vi "rosbridge.vi"(11 "ROS IP":string) -> (3 "incomming\nmessage":T1)   [LabVIEW 2013]
panel:
  out "connected?":bool
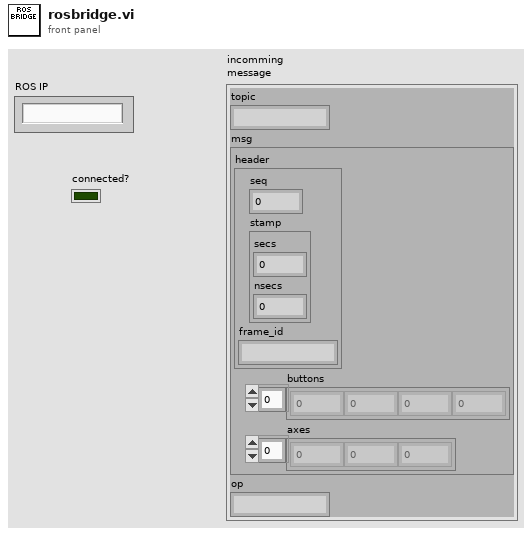
[diagram p1: front panel]
types:
  T1 = cluster{"topic":string, "msg":cluster{"header":cluster{"seq":u32, "stamp":cluster{"secs":u32, "nsecs":i32}, "frame_id":string}, "buttons":i32[], "axes":sgl[]}, "op":string}
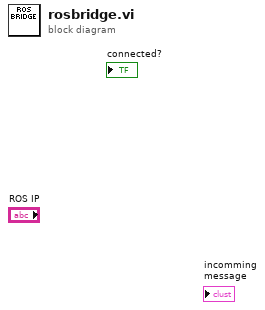
[diagram p0: block diagram]
diagram:
